vi "Write_Target_Address.vi"(8 "error in (no error)":errorcluster, 10 "Target_Address":u16 format="%x", 11 "10Bit_Address in":refnum<class "10Bit_Address.lvclass">) -> (0 "error out":errorcluster, 3 "10Bit_Address out":refnum<class "10Bit_Address.lvclass">)   [LabVIEW 2023, in "10Bit_Address.lvclass"]
uses:
  10Bit_Address/10Bit_Address.lvclass
  10Bit_Address/10Bit_Address.lvclass/10Bit_Address.ctl
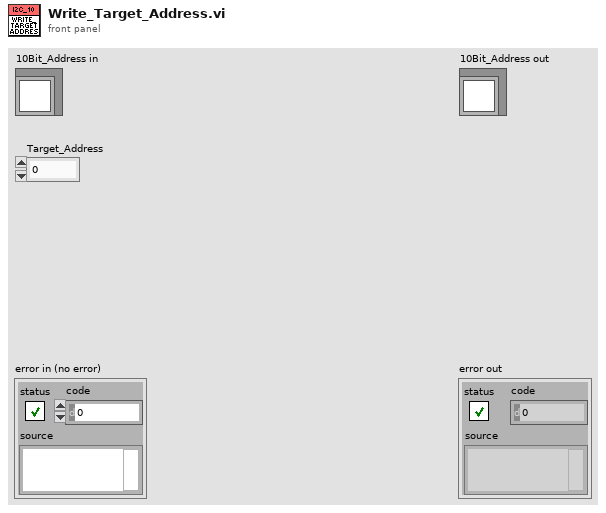
[diagram p1: front panel]
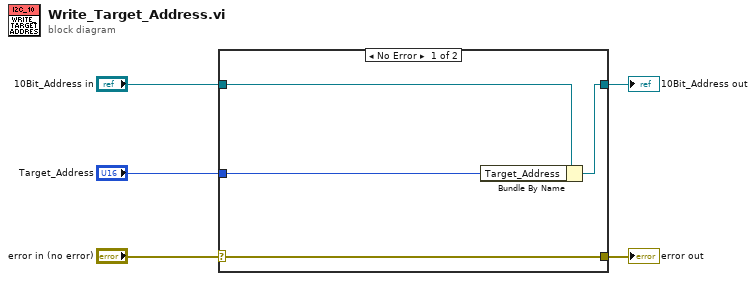
[diagram p0: block diagram]
diagram:
  n1 = case shown="No Error" "error in (no error)" {
    selector: "error in (no error)" -> [w9 w10]
    tunnel: [w9 w10] -> w4
    tunnel: [w7 w11] -> w2
    tunnel: "10Bit_Address in" -> [w8 w11]
    tunnel: "Target_Address" -> [w6 _]
    frame No Error {
      n2 = Bundle By Name(cluster=w8, "Target_Address"=w6) -> (w7:refnum<class "10Bit_Address.lvclass">)
    }
    frame Error {
    }
  }
  "error out" <- w4
  "10Bit_Address out" <- w2
